vi "MagBoard_Monitor_n64_v1.vi"() -> ()   [LabVIEW 2016]
doc: "This example performs writes and reads on a serial port, as directed by the user. You can press the Write and Read buttons, and change the Read Count, while the example is running.\n\nThe parameters set for the serial port must match the parameters of the connected instrument or device. In this example, the Read Count parameter specifies the number of bytes that the serial port reads. If there were more bytes at the port than the specified number, those bytes would not be read. If there were less bytes at the port than the specified number, you would receive a timeout error.\n\nThis example expands upon the flow control options for XON and XOFF, allowing the user to choose those control characters. Also, the user can enable or disable a termination character. Some devices require a termination character in order to identify the end of command strings. Some devices send a termination character to signify the end of data to be read. This example shows how you can end the Read operation once a termination character is detected in the buffer and/or append a termination character at the end of the Write data."
uses:
  <vilib>/Math Plots/3D Math Plots/3D Bar/3D Bar XCtrl/3D Bar.xctl
  <vilib>/Instr/_visa.llb/VISA Configure Serial Port (Instr).vi
  <vilib>/Math Plots/3D Math Plots/3D Bar/3D Bar Datatype/Public/Plot Helper (Matrix).vi
  <vilib>/Math Plots/3D Math Plots/3D Bar/3D Bar Datatype/3D Bar Datatype.lvclass
panel:
  out "Packet OK?":bool=TRUE
  in  "Tab Control":T1(tab)=enum."Basic Data"
  in  "VISA resource name":refnum<visa-resource-name>="COM11"
  in  "Serial Settings":T2={"baud rate"=115200, "data bits"=8, "parity"=enum."None", "stop bits"=10, "flow control"=0} {"flow control" items=["None"=0, "XON/XOFF"=1, "RTS/CTS"=2, "DTR/DSR"=4]; "stop bits" items=["1.0"=10, "1.5"=15, "2.0"=20]; "data bits" min=5 max=8 step=1; "baud rate" items=["75"=75, "110"=110, "134"=134, "150"=150, "300"=300, "600"=600, "1200"=1200, "1800"=1800, "2400"=2400, "4800"=4800, "7200"=7200, "9600"=9600, "14400"=14400, "19200"=19200, "28800"=28800, "38400"=38400, "56000"=56000, "57600"=57600, "115200"=115200, "128000"=128000, "230400"=230400]}
  in  "XON/XOFF Characters":T3={"XON"=enum."DC1", "XOFF"=enum."DC3"}
  in  "Termination Character":u8=10 format="%.0x"
  in  "Row LEngth":i32=8
  in  "No. Nodes":i32=64
  out "read buffer":string
  out "Serial Settings:Number of Bytes at Serial Port":u32
  out "error out":errorcluster
  out "Sensor Nodes Returned":i32=384
  in  "Node to plot":i32=4
  out "B Measure Chart":T4(graph)
  out "Time":u32=427420
  out "Sensor Readings":dbl[][](array[numeric])=[[-533.0, -111.0, 239.0], [-402.0, 166.0, 184.0], [-184.0, 154.0, 29.0], [-106.0, 74.0, 11.0], [-532.0, -109.0, 246.0], [-398.0, 164.0, 175.0], [-205.0, 152.0, 32.0], [-119.0, 65.0, 9.0], [-529.0, -110.0, 242.0], [-408.0, 166.0, 184.0], [-198.0, 158.0, 27.0], [-108.0, 61.0, 6.0], [-539.0, -106.0, 240.0], [-407.0, 158.0, 183.0], [-191.0, 156.0, 28.0], [-113.0, 73.0, 15.0], [816.0, -260.0, 842.0], [539.0, 512.0, 512.0], [156.0, 425.0, 83.0], [13.0, 142.0, -72.0], [816.0, -262.0, 840.0], [528.0, 520.0, 512.0], [162.0, 425.0, 83.0], [13.0, 137.0, -84.0], [809.0, -260.0, 840.0], [538.0, 520.0, 504.0], [162.0, 432.0, 72.0], [13.0, 136.0, -84.0], [809.0, -260.0, 846.0], [538.0, 508.0, 512.0], [158.0, 435.0, 72.0], [19.0, 136.0, -79.0], [346.0, -168.0, 14.0], [287.0, -68.0, 19.0], [161.0, -34.0, 4.0], [70.0, -44.0, -7.0], [345.0, -191.0, 19.0], [279.0, -40.0, 8.0], [167.0, -16.0, 12.0], [72.0, -23.0, 2.0], [341.0, -190.0, 17.0], [285.0, -46.0, 9.0], [149.0, -15.0, 6.0], [54.0, -40.0, -2.0], [375.0, -201.0, 19.0], [282.0, -51.0, 10.0], [135.0, -37.0, 6.0], [81.0, -57.0, -12.0], [-80.0, -193.0, -48.0], [-73.0, -136.0, -12.0], [-5.0, -122.0, -31.0], [-19.0, -118.0, -17.0], [-118.0, -187.0, -48.0], [-73.0, -115.0, -22.0], [1.0, -113.0, -27.0], [-20.0, -111.0, -8.0], [-99.0, -184.0, -40.0], [-62.0, -145.0, -17.0], [0.0, -113.0, -37.0], [-7.0, -117.0, -15.0], [-126.0, -184.0, -50.0], [-72.0, -115.0, -14.0], [-4.0, -114.0, -25.0], [-29.0, -116.0, -14.0]]
  out "3D Bar":refnum<class "3D Plot Datatype.lvclass">[](xcontrol)
  in  "Tare":bool=TRUE
  in  "Stop":bool
  # "0xA is equivalent to a '\\n' character, which is a line feed."
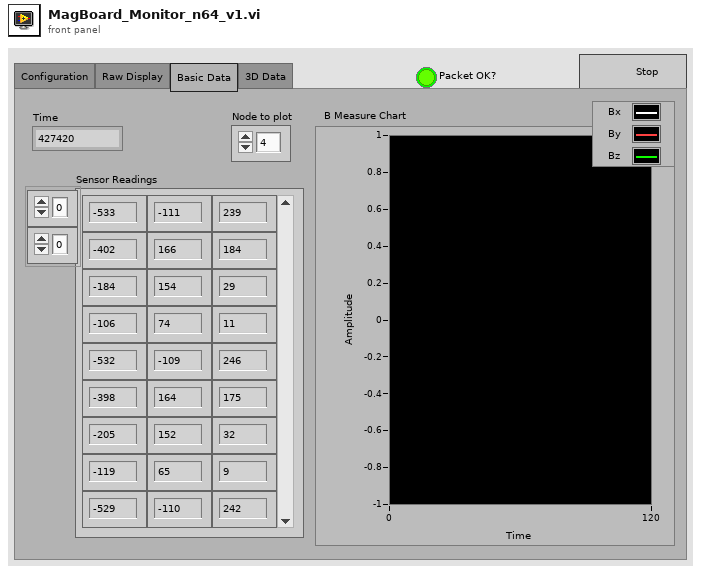
[diagram p1: front panel]
types:
  T1 = enum32{"Configuration", "Raw Display", "Basic Data", "3D Data"}
  T2 = cluster{"baud rate":u32, "data bits":u16, "parity":enum16{"None", "Odd", "Even", "Mark", "Space"}, "stop bits":u16, "flow control":u16}
  T3 = cluster{"XON":enum16{"NUL", "SOH", "STX", "ETX", "EOT", "ENQ", "ACK", "BEL", "BS", "HT", "LF", "VT", "FF", "CR", "SO", "SI", "DLE", "DC1", "DC2", "DC3", "DC4", "NAK", "SYN", "ETB", "CAN", "EM", "SUB", "ESC", "FS", "GS", "RS", "US", "SP", "!", "\"", "#", "$", "%", "&", "'", "(", ")", "*", "+", ",", "- (-)", ".", "/", "0", "1", "2", "3", "4", "5", "6", "7", "8", "9", ":", ";", "<", "=", ">", "?", "@", "A", "B", "C", "D", "E", "F", "G", "H", "I", "J", "K", "L", "M", "N", "O", "P", "Q", "R", "S", "T", "U", "V", "W", "X", "Y", "Z", "[", "\\", "]", "^", "_", "`", "a", "b", "c", "d", "e", "f", "g", "h", "i", "j", "k", "l", "m", "n", "o", "p", "q", "r", "s", "t", "u", "v", "w", "x", "y", "z", "{", "|", "}", "~"}, "XOFF":enum16{"NUL", "SOH", "STX", "ETX", "EOT", "ENQ", "ACK", "BEL", "BS", "HT", "LF", "VT", "FF", "CR", "SO", "SI", "DLE", "DC1", "DC2", "DC3", "DC4", "NAK", "SYN", "ETB", "CAN", "EM", "SUB", "ESC", "FS", "GS", "RS", "US", "SP", "!", "\"", "#", "$", "%", "&", "'", "(", ")", "*", "+", ",", "- (-)", ".", "/", "0", "1", "2", "3", "4", "5", "6", "7", "8", "9", ":", ";", "<", "=", ">", "?", "@", "A", "B", "C", "D", "E", "F", "G", "H", "I", "J", "K", "L", "M", "N", "O", "P", "Q", "R", "S", "T", "U", "V", "W", "X", "Y", "Z", "[", "\\", "]", "^", "_", "`", "a", "b", "c", "d", "e", "f", "g", "h", "i", "j", "k", "l", "m", "n", "o", "p", "q", "r", "s", "t", "u", "v", "w", "x", "y", "z", "{", "|", "}", "~"}}
  T4 = cluster{"Node XYZ List[0]":dbl, "Node XYZ List[1]":dbl, "Node XYZ List[2]":dbl}
  T5 = enum16{"NUL", "SOH", "STX", "ETX", "EOT", "ENQ", "ACK", "BEL", "BS", "HT", "LF", "VT", "FF", "CR", "SO", "SI", "DLE", "DC1", "DC2", "DC3", "DC4", "NAK", "SYN", "ETB", "CAN", "EM", "SUB", "ESC", "FS", "GS", "RS", "US", "SP", "!", "\"", "#", "$", "%", "&", "'", "(", ")", "*", "+", ",", "- (-)", ".", "/", "0", "1", "2", "3", "4", "5", "6", "7", "8", "9", ":", ";", "<", "=", ">", "?", "@", "A", "B", "C", "D", "E", "F", "G", "H", "I", "J", "K", "L", "M", "N", "O", "P", "Q", "R", "S", "T", "U", "V", "W", "X", "Y", "Z", "[", "\\", "]", "^", "_", "`", "a", "b", "c", "d", "e", "f", "g", "h", "i", "j", "k", "l", "m", "n", "o", "p", "q", "r", "s", "t", "u", "v", "w", "x", "y", "z", "{", "|", "}", "~"}
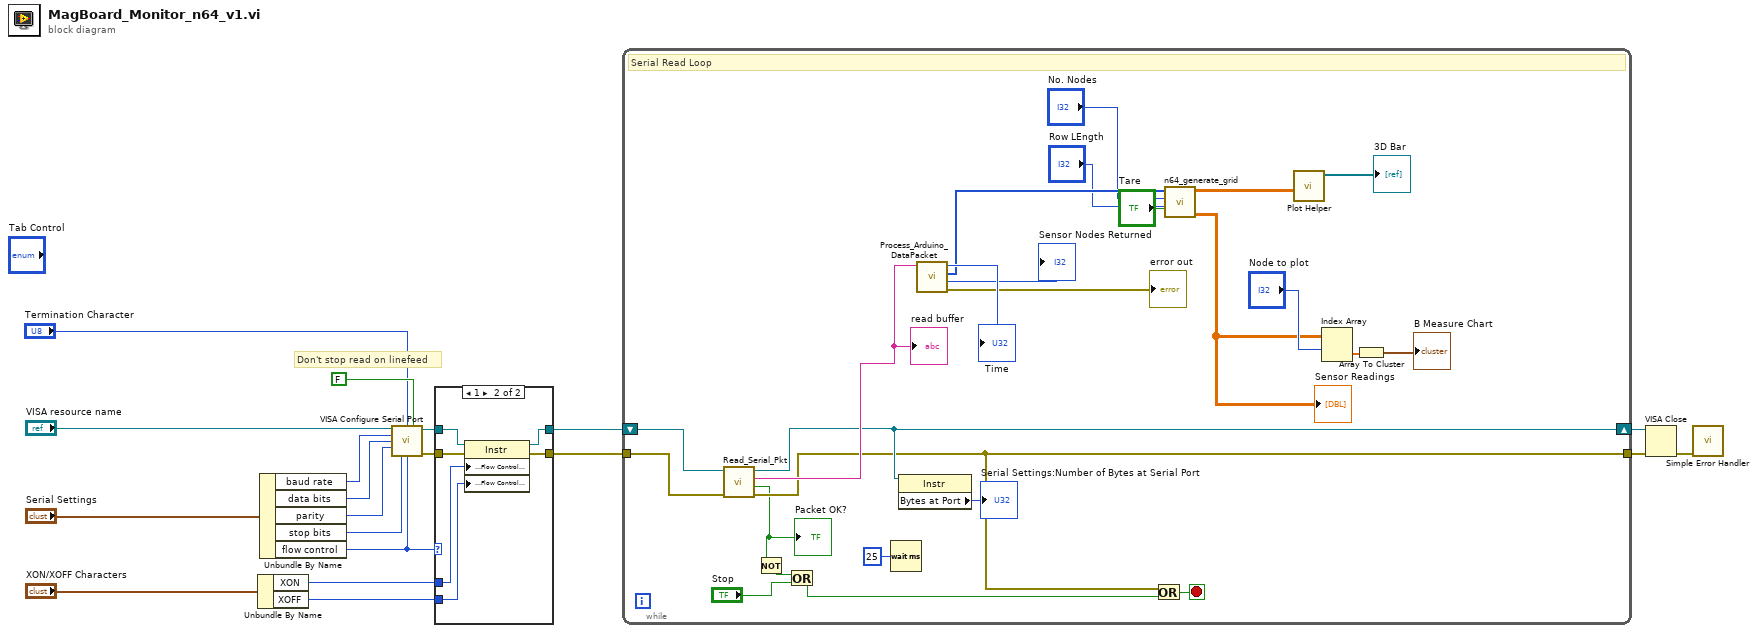
[diagram p0: block diagram]
diagram:
  # "Don't stop read on linefeed"
  n1 = Unbundle By Name("XON/XOFF Characters") -> ("XON"=w5:T5, "XOFF"=w4:T5)
  n2 = Unbundle By Name("Serial Settings") -> ("baud rate"=w12:u32, "data bits"=w13:u16, "parity"=w14:enum16{"None", "Odd", "Even", "Mark", "Space"}, "stop bits"=w15:u16, "flow control"=w6:u16)
  n3 = call-poly "VISA Configure Serial Port"("VISA resource name"="VISA resource name", "termination char\n(0xA = '\\n' = LF)"="Termination Character", "Enable Termination\nChar (T)"=FALSE ("End Read on Termination Character?"), "baud rate (9600)"=w12, "data bits (8)"=w13, "parity (0:none)"=w14, "stop bits (10: 1 bit)"=w15, "flow control (0:none)"=w6) -> ("VISA resource name out"=w16:refnum<visa-resource-name>, "error out"=w17:errorcluster)  [unwired: 2 in, 4 out]
  n4 = case shown="1" w6 {
    tunnel: [w20 w27] -> w1
    tunnel: [w21 w26] -> w2
    tunnel: w17 -> [w20 w25]
    tunnel: w16 -> [w21 w24]
    tunnel: w5 -> [_ w23]
    tunnel: w4 -> [_ w22]
    frame Default {
    }
    frame 1 {
      n5 = property class="Instr"(reference=w24, error in=w25, "Serial Settings:Flow Control XON Character"=w23, "Serial Settings:Flow Control XOFF Character"=w22) -> (reference out=w26:refnum<visa-resource-name>, error out=w27:errorcluster)
    }
  }
  n6 = while {
    shift-right: [w44] -> w7
    shift-left: w2 -> [w46]
    tunnel: w1 -> [w47]
    tunnel: [w43] -> w8
    stop <- w51 stop-if-true
    # "Serial Read Loop"
    n7 = call "Read_Serial_Pkt.vi"("error in"=w47, "VISA resource in"=w46) -> ("error out"=w43:errorcluster, "Packet OK?"=w41:bool, "Data"=w45:string, "VISA resource out"=w44:refnum<visa-resource-name>)  [unwired: 6 in]
    "read buffer" <- w45
    "Packet OK?" <- w41
    n8 = Not(x=w41) -> (.not. x?=w38:bool)
    n9 = Or(x=w38, y="Stop") -> (x .or. y?=w39:bool)
    n10 = Wait (ms)(milliseconds to wait=u32 25) -> ()  [unwired: 1 out]
    n11 = property class="Instr"(reference=w44) -> ("Bytes at Port"=→"Serial Settings:Number of Bytes at Serial Port":u32)  [unwired: 1 in, 2 out]
    n12 = call "Process_Arduino_DataPacket.vi"("Data Packet"=w45) -> ("error out"=→"error out":errorcluster, "Sensor Packets Returned"=→"Sensor Nodes Returned":i32, "Sensor Readings (Signed)"=w34:i16[], "Time"=→"Time":u32)  [unwired: 7 in]
    n13 = Or(x=w43, y=w39) -> (x .or. y?=w51:bool)
    n14 = call "n64_generate_grid.vi"("Tare"="Tare", "Row Length"="Row LEngth", "No. Nodes"="No. Nodes", "Sensor Readings (PACKET)"=w34) -> ("Node XYZ List"=w33:dbl[][], "Z (GRID)"=w36:dbl[][])  [unwired: 4 in, 2 out]
    "Sensor Readings" <- w33
    n15 = call-poly <vilib>:"Plot Helper.vi"("z matrix"=w36) -> ("3D Plot lvclass Array out"=→"3D Bar":refnum<class "3D Plot Datatype.lvclass">[])  [unwired: 2 in, 8 out]
    n16 = Index Array(array=w33, index (row)="Node to plot") -> (element=w32:dbl[])  [unwired: 1 in]
    n17 = Array To Cluster(array=w32) -> (cluster=→"B Measure Chart":T4)
  }
  n18 = VISA Close(VISA resource name=w7, error in (no error)=w8) -> (error out=w9:errorcluster)
  n19 = call <vilib>:"Simple Error Handler.vi"("error in (no error)"=w9) -> ()  [unwired: 1 in, 8 out]
